vi "Create APU Tree Layout - Multi FPGA.vi"(8 "error in (no error)":errorcluster, 9 "rio name":string, 10 "engine name":string, 11 "Section Ptr":T1 format="%.0x") -> (0 "error out":errorcluster, 2 "APU ref":T1 format="%.0x", 3 "Section Ptr dup":T1 format="%.0x")   [LabVIEW 2017, in "Engine Simulation Toolkit System Explorer.lvlib"]
uses:
  Engine Simulation Toolkit System Explorer.lvlib
  <vilib>/NI Veristand/Custom Device API/Custom Device Item Ref.ctl
  <vilib>/NI Veristand/Custom Device API/Custom Device Channel Type.ctl
  Shared/Constants and GUIDs.vi
  Shared/Properties.vi
  <vilib>/NI Veristand/Custom Device API/Set Item Property (String).vi
  <vilib>/NI Veristand/Custom Device API/Custom Device API.lvlib
  Shared/Engine Simulation Toolkit Shared.lvlib
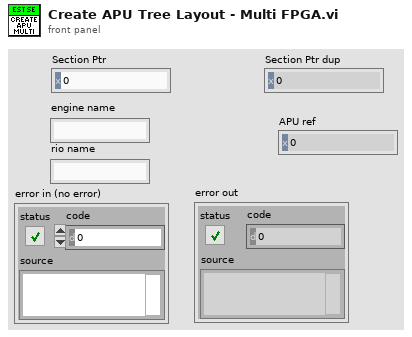
[diagram p1: front panel]
types:
  T1 = typedef "Custom Device API.lvlib/Custom Device Item Ref.ctl" = u64
  T2 = typedef "Custom Device API.lvlib/Custom Device Channel Type.ctl" = enum16{"Input", "Output"}
  T3 = typedef "Engine Simulation Toolkit Shared.lvlib/Channel.ctl" = cluster{"Name":string, "Units":string, "Default":dbl, "Description":string, "Scalable":bool}
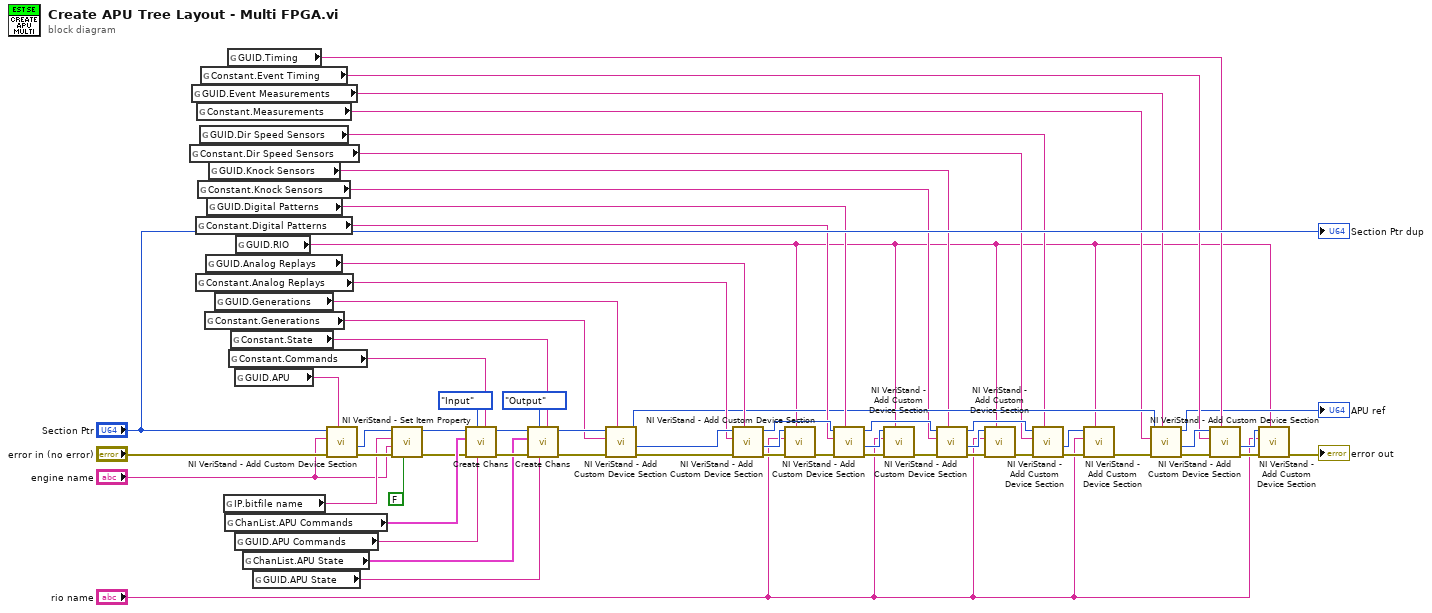
[diagram p0: block diagram]
diagram:
  n1 = global read "Constants and GUIDs.vi" "Constant.Dir Speed Sensors"() -> (w17:string)
  n2 = global read "Constants and GUIDs.vi" "GUID.Event Measurements"() -> (w33:string)
  n3 = global read "Constants and GUIDs.vi" "Constant.Digital Patterns"() -> (w39:string)
  n4 = global read "Constants and GUIDs.vi" "Constant.Analog Replays"() -> (w42:string)
  n5 = global read "Constants and GUIDs.vi" "Constant.Measurements"() -> (w36:string)
  n6 = global read "Constants and GUIDs.vi" "Constant.Knock Sensors"() -> (w21:string)
  n7 = global read "Constants and GUIDs.vi" "GUID.Dir Speed Sensors"() -> (w18:string)
  n8 = global read "Constants and GUIDs.vi" "Constant.Event Timing"() -> (w32:string)
  n9 = global read "Constants and GUIDs.vi" "Constant.Generations"() -> (w46:string)
  n10 = global read "Constants and GUIDs.vi" "GUID.Analog Replays"() -> (w41:string)
  n11 = global read "Constants and GUIDs.vi" "GUID.Digital Patterns"() -> (w38:string)
  n12 = global read "Constants and GUIDs.vi" "GUID.Knock Sensors"() -> (w22:string)
  n13 = global read "Constants and GUIDs.vi" "GUID.Generations"() -> (w45:string)
  n14 = global read "Properties.vi" "IP.bitfile name"() -> (w29:string)
  n15 = global read "Constants and GUIDs.vi" "ChanList.APU Commands"() -> (w56:T3[])
  n16 = global read "Constants and GUIDs.vi" "GUID.Timing"() -> (w31:string)
  n17 = global read "Constants and GUIDs.vi" "Constant.Commands"() -> (w57:string)
  n18 = global read "Constants and GUIDs.vi" "Constant.State"() -> (w51:string)
  n19 = global read "Constants and GUIDs.vi" "GUID.APU"() -> (w61:string)
  n20 = global read "Constants and GUIDs.vi" "GUID.APU Commands"() -> (w48:string)
  n21 = global read "Constants and GUIDs.vi" "GUID.RIO"() -> (w4:string)
  n22 = global read "Constants and GUIDs.vi" "ChanList.APU State"() -> (w53:T3[])
  n23 = global read "Constants and GUIDs.vi" "GUID.APU State"() -> (w47:string)
  n24 = call <vilib>:"NI VeriStand - Add Custom Device Section.vi"("GUID (Default Section)"=w61, "error in (no error)"="error in (no error)", "Section Name"="engine name", "Parent Ref in"="Section Ptr") -> ("error out"=w59:errorcluster, "Section Ptr"=w30:T1)  [unwired: 4 in, 2 out]
  n25 = call-poly <vilib>:"NI VeriStand - Set Item Property.vi"("Binary String (T)"=FALSE, "error in (no error)"=w59, "Value"="engine name", "Property Name"=w29, "Item Ref in"=w30) -> ("error out"=w2:errorcluster, "Item Ref out"=w1:T1)  [unwired: 4 in, 1 out]
  n26 = call "Create Chans.vi"("New Section Name (none)"=w57, "new section GUID (\"\":del prot)"=w48, "Type"=Custom_Device_Channel_Type."Input", "error in (no error)"=w2, "Channels"=w56, "Section Ptr"=w1) -> ("error out"=w55:errorcluster, "Section Ptr dup"=w54:T1)  [unwired: 2 in, 2 out]
  n27 = call "Create Chans.vi"("New Section Name (none)"=w51, "new section GUID (\"\":del prot)"=w47, "Type"=Custom_Device_Channel_Type."Output", "error in (no error)"=w55, "Channels"=w53, "Section Ptr"=w54) -> ("error out"=w50:errorcluster, "Section Ptr dup"=w49:T1)  [unwired: 2 in, 2 out]
  n28 = call <vilib>:"NI VeriStand - Add Custom Device Section.vi"("GUID (Default Section)"=w45, "error in (no error)"=w50, "Section Name"=w46, "Parent Ref in"=w49) -> ("error out"=w44:errorcluster, "Section Ptr"=w43:T1, "Parent Ref out"=w37:T1)  [unwired: 4 in, 1 out]
  n29 = call <vilib>:"NI VeriStand - Add Custom Device Section.vi"("GUID (Default Section)"=w41, "error in (no error)"=w44, "Section Name"=w42, "Parent Ref in"=w43) -> ("error out"=w16:errorcluster, "Section Ptr"=w14:T1, "Parent Ref out"=w40:T1)  [unwired: 4 in, 1 out]
  n30 = call <vilib>:"NI VeriStand - Add Custom Device Section.vi"("GUID (Default Section)"=w4, "error in (no error)"=w16, "Section Name"="rio name", "Parent Ref in"=w14) -> ("error out"=w15:errorcluster)  [unwired: 4 in, 3 out]
  n31 = call <vilib>:"NI VeriStand - Add Custom Device Section.vi"("GUID (Default Section)"=w38, "error in (no error)"=w15, "Section Name"=w39, "Parent Ref in"=w40) -> ("error out"=w25:errorcluster, "Section Ptr"=w12:T1, "Parent Ref out"=w24:T1)  [unwired: 4 in, 1 out]
  n32 = call <vilib>:"NI VeriStand - Add Custom Device Section.vi"("GUID (Default Section)"=w4, "error in (no error)"=w25, "Section Name"="rio name", "Parent Ref in"=w12) -> ("error out"=w13:errorcluster)  [unwired: 4 in, 3 out]
  n33 = call <vilib>:"NI VeriStand - Add Custom Device Section.vi"("GUID (Default Section)"=w22, "error in (no error)"=w13, "Section Name"=w21, "Parent Ref in"=w24) -> ("error out"=w23:errorcluster, "Section Ptr"=w10:T1, "Parent Ref out"=w19:T1)  [unwired: 4 in, 1 out]
  n34 = call <vilib>:"NI VeriStand - Add Custom Device Section.vi"("GUID (Default Section)"=w4, "error in (no error)"=w23, "Section Name"="rio name", "Parent Ref in"=w10) -> ("error out"=w11:errorcluster)  [unwired: 4 in, 3 out]
  n35 = call <vilib>:"NI VeriStand - Add Custom Device Section.vi"("GUID (Default Section)"=w18, "error in (no error)"=w11, "Section Name"=w17, "Parent Ref in"=w19) -> ("error out"=w20:errorcluster, "Section Ptr"=w8:T1)  [unwired: 4 in, 2 out]
  n36 = call <vilib>:"NI VeriStand - Add Custom Device Section.vi"("GUID (Default Section)"=w4, "error in (no error)"=w20, "Section Name"="rio name", "Parent Ref in"=w8) -> ("error out"=w9:errorcluster)  [unwired: 4 in, 3 out]
  n37 = call <vilib>:"NI VeriStand - Add Custom Device Section.vi"("GUID (Default Section)"=w33, "error in (no error)"=w9, "Section Name"=w36, "Parent Ref in"=w37) -> ("error out"=w35:errorcluster, "Section Ptr"=w34:T1, "Parent Ref out"=→"APU ref":T1)  [unwired: 4 in, 1 out]
  n38 = call <vilib>:"NI VeriStand - Add Custom Device Section.vi"("GUID (Default Section)"=w31, "error in (no error)"=w35, "Section Name"=w32, "Parent Ref in"=w34) -> ("error out"=w7:errorcluster, "Section Ptr"=w5:T1)  [unwired: 4 in, 2 out]
  n39 = call <vilib>:"NI VeriStand - Add Custom Device Section.vi"("GUID (Default Section)"=w4, "error in (no error)"=w7, "Section Name"="rio name", "Parent Ref in"=w5) -> ("error out"=→"error out":errorcluster)  [unwired: 4 in, 3 out]
  "Section Ptr dup" <- "Section Ptr"
